vi "Motion_Wait for Gantry Move.vi"(8 "error in (no error)":errorcluster, 10 "Timeout sec (-1 = No timeout)":i32=-1, 11 "TCP Connection Refnum in":refnum<k5>) -> (0 "error out":errorcluster, 1 "Time Elapsed":dbl, 2 "Timed Out?":bool, 3 "TCP Connection Refnum (dup)":refnum<k5>)   [LabVIEW 2010]
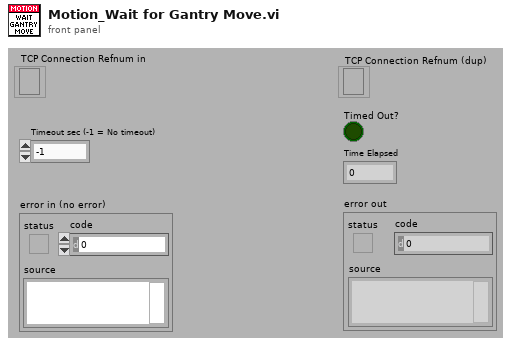
[diagram p1: front panel]
types:
  T1 = cluster{"Gantry Enabled":bool, "Gantry Power Error":bool, "Gantry Moving":bool, "Gantry At Position":bool, "Gantry Goto Error":bool, "Gantry Goto Aborted":bool, "Gantry Homing":bool, "Gantry Home Error":bool, "Gantry Home Required":bool, "Gantry Home Aborted":bool, "Gantry General Alarm":bool, "Motion Alarm":bool}
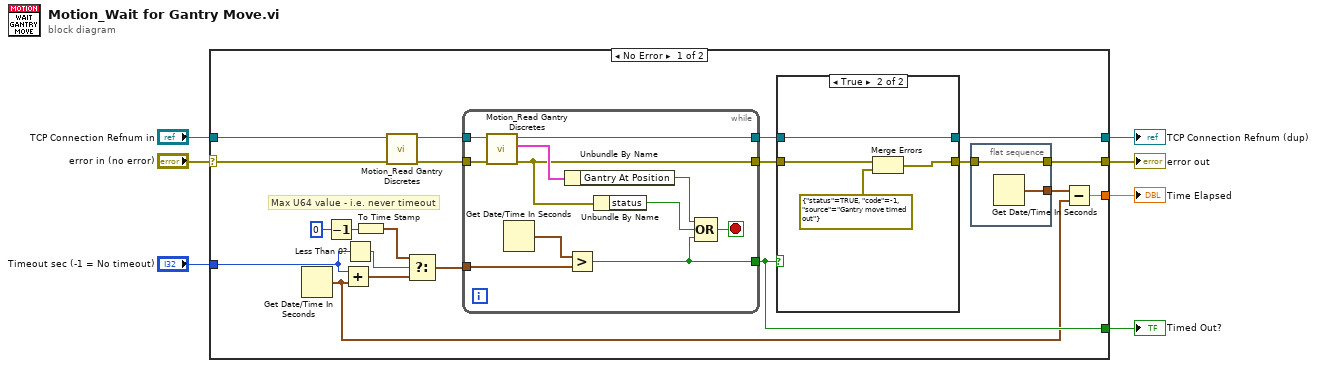
[diagram p0: block diagram]
diagram:
  n1 = case shown="No Error" "error in (no error)" {
    selector: "error in (no error)" -> [w19 w47]
    tunnel: "Timeout sec (-1 = No timeout)" -> [w14 _]
    tunnel: "TCP Connection Refnum in" -> [w17 w48]
    tunnel: [w11 w47] -> w4
    tunnel: [w15 w48] -> w3
    tunnel: [w13 _] -> w2
    tunnel: [w8 _] -> w1
    frame No Error {
      # "Max U64 value - i.e. never timeout"
      n2 = Get Date/Time In Seconds() -> (seconds since 1Jan1904=w9:timestamp)
      n3 = Decrement(x=u64 0) -> (x-1=w25:u64)
      n4 = Add(x=w14, y=w9) -> (x+y=w23:timestamp)
      n5 = Less Than 0?(x=w14) -> (x < 0?=w27:bool)
      n6 = To Time Stamp(1:w25) -> (0:w24:timestamp)
      n7 = call "Motion_Read Gantry Discretes.vi"("error in (no error)"=w19, "TCP Connection Refnum in"=w17) -> ("error out"=w18:errorcluster, "TCP Connection Refnum (dup)"=w16:refnum<k5>)  [unwired: 7 in, 1 out]
      n8 = Select(t=w24, s=w27, f=w23) -> (s? t:f=w22:timestamp)
      n9 = while {
        tunnel: [w46] -> w20
        tunnel: [w39] -> w21
        tunnel: w22 -> [w42]
        tunnel: [w40] -> w13
        tunnel: w18 -> [w37]
        tunnel: w16 -> [w36]
        stop <- w41 stop-if-true
        n10 = call "Motion_Read Gantry Discretes.vi"("error in (no error)"=w37, "TCP Connection Refnum in"=w36) -> ("error out"=w39:errorcluster, "Gantry Discretes"=w45:T1, "TCP Connection Refnum (dup)"=w46:refnum<k5>)  [unwired: 7 in]
        n11 = Get Date/Time In Seconds() -> (seconds since 1Jan1904=w43:timestamp)
        n12 = Unbundle By Name(w45) -> ("Gantry At Position"=w44:bool)
        n13 = Greater?(x=w43, y=w42) -> (0:w40:bool)
        n14 = Unbundle By Name(w39) -> ("status"=w38:bool)
        n15 = Compound Arithmetic op=OR(w44, w38, w40) -> (w41:bool)
      }
      n16 = case shown="True" w13 {
        tunnel: w21 -> [w31 w35]
        tunnel: w20 -> [w30 w32]
        tunnel: [w31 w33] -> w12
        tunnel: [w30 w32] -> w15
        frame False {
        }
        frame True {
          n17 = Merge Errors(w35, errorcluster {"status"=TRUE, "code"=-1, "source"="Gantry move timed out"} ("error in")) -> (w33:errorcluster)
        }
      }
      n18 = flat-sequence {
        tunnel: w12 -> [w29]
        tunnel: [w29] -> w11
        tunnel: [w28] -> w10
        frame #0 {
          n19 = Get Date/Time In Seconds() -> (seconds since 1Jan1904=w28:timestamp)
        }
      }
      n20 = Subtract(x=w10, y=w9) -> (x-y=w8:dbl)
    }
    frame Error {
    }
  }
  "error out" <- w4
  "TCP Connection Refnum (dup)" <- w3
  "Timed Out?" <- w2
  "Time Elapsed" <- w1
